vi "NXT the tug main.vi"() -> ()   [LabVIEW 2012, in "ENGR3390 Tug Boat.lvrbt"]
uses:
  ENGR3390 Tug Boat.lvrbt
  <vilib>/NXT/Block Support/NXT_InputPort.ctl
  <vilib>/NXT/Dual Mode Library/Display/drawText.vi
  <vilib>/NXT/Dual Mode Library/Sound/Tone.vi
panel:
  out "End\nIndex":i32=9
  out "Start\nIndex":i32=6
  out "Dist Array":i16[](array[numeric])
  out "IR Index":u16
  out "Dist":i16
  out "error out":errorcluster
  out "FB array":i16[](array[numeric])=[7, 8, 6, 9, 5, 10, 4, 11, 3, 12, 2, 13, 1, 14, 0, 15]
  out "Tug A":i16[](array[numeric])=[7, 8, 6, 9, 5, 10, 4, 11, 3, 12, 2, 13, 1, 14, 0, 15]
  out "FB V":i16
  out "FB H":i16
  out "Mode":i16
  out "String from PC":string
  out "Return":string
  out "Motor":u16
  out "Rudder":u16
  out "Bvolts":i32
  in  "stop":bool
  # "This is the main vi for the tug NXT code."
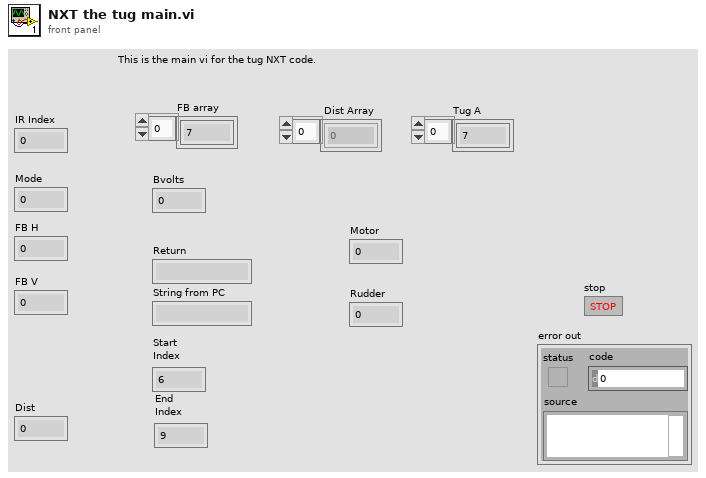
[diagram p1: front panel]
types:
  T1 = cluster{"Servo Number":u8, "Position":u16, "Speed":u8}
  T2 = typedef "NXT_InputPort.ctl" = u8
  T3 = typedef "LVHSConnector.ctl" = cluster{"Hardware":string, "Flattened String":string}
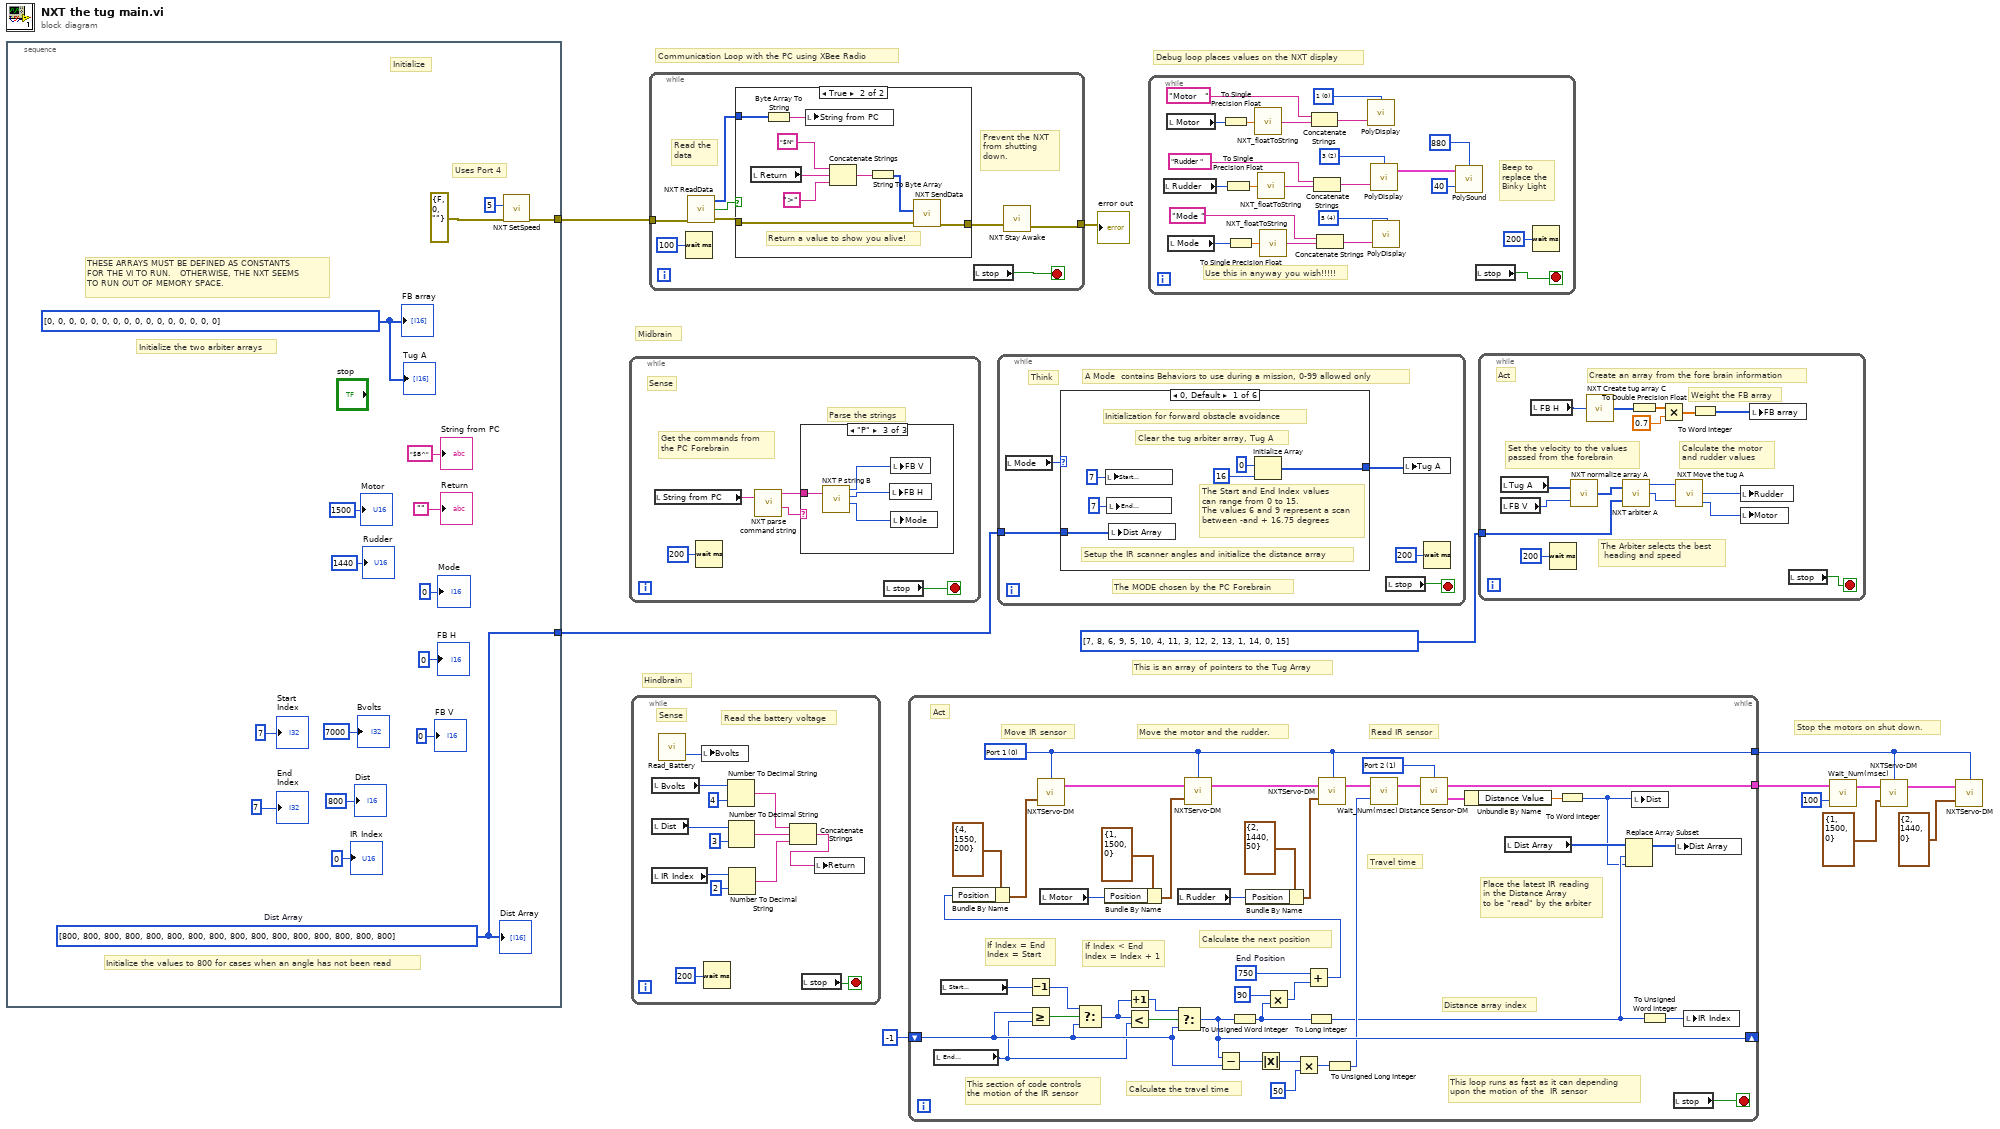
[diagram p0: block diagram]
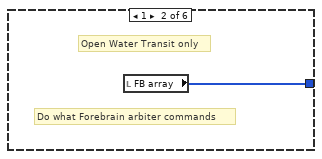
[diagram p3: hidden frame]
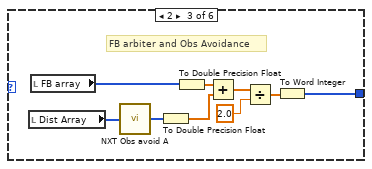
[diagram p4: hidden frame]
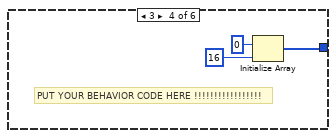
[diagram p5: hidden frame]
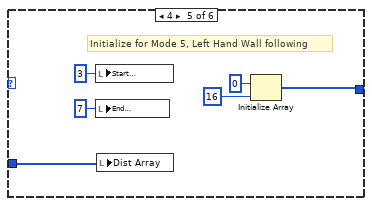
[diagram p6: hidden frame]
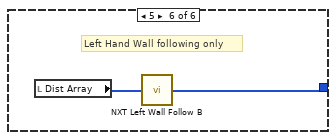
[diagram p7: hidden frame]
diagram:
  # "Debug loop places values on the NXT display"
  # "Communication Loop with the PC using XBee Radio"
  # "Stop the motors on shut down."
  # "This is an array of pointers to the Tug Array"
  # "Hindbrain"
  # "Midbrain"
  n1 = stacked-sequence {
    tunnel: [w19] -> w11
    tunnel: [w15] -> w1
    frame #0 {
      w15 = i16[] [800, 800, 800, 800, 800, 800, 800, 800, 800, 800, 800, 800, 800, 800, 800, 800]  # Dist Array
      w18 = i16[] [0, 0, 0, 0, 0, 0, 0, 0, 0, 0, 0, 0, 0, 0, 0, 0] ("Array angle\npointers")
      # "Initialize the two arbiter arrays"
      # "Initialize the values to 800 for cases when an angle has not been read"
      # "THESE ARRAYS MUST BE DEFINED AS CONSTANTS\nFOR THE VI TO RUN.   OTHERWISE, THE NXT SEEMS \nTO RUN OUT OF MEMORY SPACE."
      # "Uses Port 4"
      # "Initialize"
      n2 = call "NXT SetSpeed.vi"("error in (no error)"=errorcluster {"status"=FALSE, "code"=0, "source"=""} ("error out"), "Speed"=u8 5) -> ("error out"=w19:errorcluster)  [unwired: 5 in]
      "Bvolts" <- 7000 ("Bvolts")
      "Rudder" <- u16 1440 ("Bvolts")
      "Motor" <- u16 1500 ("Bvolts")
      "Return" <- "" ("Empty String Constant")
      "String from PC" <- "$B^" ("String from PC")
      "Mode" <- i16 0 ("Mode")
      "FB H" <- i16 0 ("Target\nHeading")
      "FB V" <- i16 0 ("Target\nHeading")
      "Tug A" <- w18
      "FB array" <- w18
      "IR Index" <- u16 0 ("IR Index")
      "Dist" <- i16 800 ("Dist")
      "Dist Array" <- w15
      "End\nIndex" <- 7 ("End\nIndex")
      "Start\nIndex" <- 7 ("Start\nIndex")
    }
  }
  n3 = while {
    stop <- w34 stop-if-true
    # "Get the commands from\nthe PC Forebrain"
    # "Parse the strings"
    # "Sense"
    n4 = local read "String from PC"() -> (w33:string)
    n5 = Wait (ms)(milliseconds to wait=u32 200) -> ()  [unwired: 1 out]
    n6 = call "NXT parse command string.vi"("String"=w33) -> ("Remaining\nString"=w31:string, "Command"=w32:string)  [unwired: 1 in, 2 out]
    n7 = case shown="\"P\"" w32 {
      tunnel: w31 -> [_ _ w35]
      frame Default {
      }
      frame "B" {
        # "Do nothing"
      }
      frame "P" {
        n8 = call "NXT P string B.vi"("string"=w35) -> ("Desired Velocity"=w38:i16, "Local Heading"=w37:i16, "Mode"=w36:i16)  [unwired: 1 in, 1 out]
        n9 = local write "FB H"(w37) -> ()
        n10 = local write "FB V"(w38) -> ()
        n11 = local write "Mode"(w36) -> ()
      }
    }
    n12 = local read "stop"() -> (w34:bool)
  }
  n13 = while {
    stop <- w51 stop-if-true
    # "Read the battery voltage"
    # "Sense"
    n14 = local read "Bvolts"() -> (w47:i32)
    n15 = local read "Dist"() -> (w46:i16)
    n16 = local read "IR Index"() -> (w44:u16)
    n17 = call <vilib>:"Read_Battery.vi"() -> ("millivolts"=w50:i32)  [unwired: 3 in, 1 out]
    n18 = local write "Bvolts"(w50) -> ()
    n19 = Wait (ms)(milliseconds to wait=u32 200) -> ()  [unwired: 1 out]
    n20 = Number To Decimal String(number=w47, width (-)=i16 4) -> (decimal integer string=w41:string)
    n21 = Number To Decimal String(number=w46, width (-)=i16 3) -> (decimal integer string=w42:string)
    n22 = Number To Decimal String(number=w44, width (-)=i16 2) -> (decimal integer string=w40:string)
    n23 = Concatenate Strings(w41, w42, w40) -> (w39:string)
    n24 = local read "stop"() -> (w51:bool)
    n25 = local write "Return"(w39) -> ()
  }
  n26 = while {
    tunnel: w11 -> [w58]
    tunnel: [w52] -> w10
    stop <- w56 stop-if-true
    # "Prevent the NXT\nfrom shutting \ndown."
    # "Read the \ndata"
    n27 = Wait (ms)(milliseconds to wait=u32 100) -> ()  [unwired: 1 out]
    n28 = call "NXT ReadData.vi"("error in (no error)"=w58) -> ("error out"=w59:errorcluster, "Valid String?"=w57:bool, "Data Out"=w55:u8[])  [unwired: 3 in]
    n29 = case shown="True" w57 {
      tunnel: [w60 w63] -> w53
      tunnel: w59 -> [w60 w68]
      tunnel: w55 -> [_ w61]
      frame False {
        # "Data is not valid\ndo nothing"
      }
      frame True {
        # "Return a value to show you alive!"
        n30 = local read "Return"() -> (w64:string)
        n31 = Byte Array To String(unsigned byte array=w61) -> (string=w62:string)
        n32 = local write "String from PC"(w62) -> ()
        n33 = Concatenate Strings("$N" ("string"), w64, ">" ("string")) -> (w65:string)
        n34 = String To Byte Array(string=w65) -> (unsigned byte array=w69:u8[])
        n35 = call "NXT SendData.vi"("error in (no error)"=w68, "Data"=w69) -> ("error out"=w63:errorcluster)  [unwired: 7 in]
      }
    }
    n36 = local read "stop"() -> (w56:bool)
    n37 = call "NXT Stay Awake.vi"("error in (no error)"=w53) -> ("error out"=w52:errorcluster)  [unwired: 2 in]
  }
  "error out" <- w10
  n38 = while {
    shift-right: [w87] -> _
    shift-left: -1 -> [w88]
    tunnel: [w80] -> w5
    tunnel: [w81] -> w4
    stop <- w104 stop-if-true
    w93 = u16 750  # End Position
    w100 = T2 1 items=["Port 1", "Port 2", "Port 3", "Port 4"] ("Input Port")
    w81 = T2 0 items=["Port 1", "Port 2", "Port 3", "Port 4"] ("Input Port")
    # "Place the latest IR reading\nin the Distance Array\nto be \"read\" by the arbiter"
    # "Distance array index"
    # "This loop runs as fast as it can depending\nupon the motion of the  IR sensor"
    # "Travel time"
    # "This section of code controls\nthe motion of the IR sensor"
    # "Calculate the next position"
    # "Calculate the travel time"
    # "If Index = End\nIndex = Start"
    # "If Index < End\nIndex = Index + 1"
    # "Read IR sensor"
    # "Move IR sensor"
    # "Move the motor and the rudder."
    # "Act"
    n39 = local read "End\nIndex"() -> (w73:i32)
    n40 = local read "Start\nIndex"() -> (w74:i32)
    n41 = Decrement(x=w74) -> (x-1=w75:i32)
    n42 = Greater Or Equal?(x=w88, y=w73) -> (x >= y?=w91:bool)
    n43 = local read "Motor"() -> (w105:u16)
    n44 = Select(t=w75, s=w91, f=w88) -> (s? t:f=w92:i32)
    n45 = Bundle By Name(cluster=T1 {"Servo Number"=1, "Position"=1500, "Speed"=0} ("Input of NXTServo"), "Position"=w105) -> (w108:T1)
    n46 = Increment(x=w92) -> (x+1=w89:i32)
    n47 = Less?(x=w92, y=w73) -> (x < y?=w90:bool)
    n48 = Select(t=w89, s=w90, f=w88) -> (s? t:f=w87:i32)
    n49 = local read "Rudder"() -> (w106:u16)
    n50 = Subtract(x=w87, y=w88) -> (x-y=w96:i32)
    n51 = To Unsigned Word Integer(number=w87) -> (unsigned 16bit integer=w79:u16)
    n52 = Bundle By Name(cluster=T1 {"Servo Number"=2, "Position"=1440, "Speed"=50} ("Input of NXTServo"), "Position"=w106) -> (w111:T1)
    n53 = Absolute Value(x=w96) -> (abs(x)=w97:i32)
    n54 = Multiply(x=u16 90, y=w79) -> (x*y=w95:u16)
    n55 = Multiply(x=w97, y=50) -> (x*y=w84:i32)
    n56 = Add(x=w93, y=w95) -> (x+y=w82:u16)
    n57 = Bundle By Name(cluster=T1 {"Servo Number"=4, "Position"=1550, "Speed"=200} ("Input of NXTServo"), "Position"=w82) -> (w103:T1)
    n58 = call "NXTServo-DM.vi"("Input of NXTServo"=w103, "Input Port"=w81) -> ("NXT dup"=w101:T3)  [unwired: 1 in, 1 out]
    n59 = call "NXTServo-DM.vi"("Input of NXTServo"=w108, "NXT"=w101, "Input Port"=w81) -> ("NXT dup"=w107:T3)  [unwired: 1 out]
    n60 = To Long Integer(number=w79) -> (32bit integer=w72:i32)
    n61 = call "NXTServo-DM.vi"("Input of NXTServo"=w111, "NXT"=w107, "Input Port"=w81) -> ("NXT dup"=w86:T3)  [unwired: 1 out]
    n62 = To Unsigned Long Integer(number=w84) -> (unsigned 32bit integer=w83:u32)
    n63 = call <vilib>:"Wait_Num(msec).vi"("Time (100 msec)"=w83, "NXT"=w86) -> ("NXT"=w85:T3)  [unwired: 2 in]
    n64 = call "Distance Sensor-DM.vi"("NXT"=w85, "Input Port"=w100) -> ("Output of Distance Sensor"=w99:cluster{"Distance Value":ext, "Status":bool}, "NXT dup"=w80:T3)  [unwired: 1 in]
    n65 = Unbundle By Name(w99) -> ("Distance Value"=w78:ext)
    n66 = local read "Dist Array"() -> (w77:i16[])
    n67 = To Word Integer(number=w78) -> (16bit integer=w70:i16)
    n68 = Replace Array Subset(array=w77, new element=w70, index=w72) -> (w76:i16[])
    n69 = local write "Dist"(w70) -> ()
    n70 = To Unsigned Word Integer(number=w72) -> (unsigned 16bit integer=w71:u16)
    n71 = local read "stop"() -> (w104:bool)
    n72 = local write "Dist Array"(w76) -> ()
    n73 = local write "IR Index"(w71) -> ()
  }
  n74 = while {
    tunnel: w1 -> [w112]
    stop <- w116 stop-if-true
    # "The MODE chosen by the PC Forebrain"
    # "A Mode  contains Behaviors to use during a mission, 0-99 allowed only"
    # "Think"
    n75 = local read "Mode"() -> (w115:i16)
    n76 = case shown="0, Default" w115 {
      tunnel: [w120 w123 w125 w133 w136 w142] -> w114
      tunnel: w112 -> [w119 _ _ _ w139 _]
      frame 0, Default {
        # "The Start and End Index values \ncan range from 0 to 15.\nThe values 6 and 9 represent a scan\nbetween -and + 16.75 degrees"
        # "Setup the IR scanner angles and initialize the distance array"
        # "Clear the tug arbiter array, Tug A"
        # "Initialization for forward obstacle avoidance"
        n77 = local write "Start\nIndex"(7 ("Start\nIndex")) -> ()
        n78 = local write "End\nIndex"(7 ("End\nIndex")) -> ()
        n79 = local write "Dist Array"(w119) -> ()
        n80 = Initialize Array(i16 0 ("element"), 16 ("dimension size")) -> (w120:i16[])
      }
      frame 1 {
        # "Open Water Transit only"
        # "Do what Forebrain arbiter commands"
        n81 = local read "FB array"() -> (w123:i16[])
      }
      frame 2 {
        # "FB arbiter and Obs Avoidance"
        n82 = local read "Dist Array"() -> (w124:i16[])
        n83 = local read "FB array"() -> (w128:i16[])
        n84 = call "NXT Obs avoid A.vi"("Distance array"=w124) -> ("Obs array"=w127:i16[])
        n85 = To Double Precision Float(number=w127) -> (double precision float=w126:dbl[])
        n86 = To Double Precision Float(number=w128) -> (double precision float=w132:dbl[])
        n87 = Add(x=w132, y=w126) -> (x+y=w131:dbl[])
        n88 = Divide(x=w131, y=2.0) -> (x/y=w129:dbl[])
        n89 = To Word Integer(number=w129) -> (16bit integer=w125:i16[])
      }
      frame 3 {
        # "PUT YOUR BEHAVIOR CODE HERE !!!!!!!!!!!!!!!!!"
        n90 = Initialize Array(i16 0 ("element"), 16 ("dimension size")) -> (w133:i16[])
      }
      frame 4 {
        # "Initialize for Mode 5, Left Hand Wall following"
        n91 = local write "Start\nIndex"(3 ("Start\nIndex")) -> ()
        n92 = local write "End\nIndex"(7 ("End\nIndex")) -> ()
        n93 = local write "Dist Array"(w139) -> ()
        n94 = Initialize Array(i16 0 ("element"), 16 ("dimension size")) -> (w136:i16[])
      }
      frame 5 {
        # "Left Hand Wall following only"
        n95 = local read "Dist Array"() -> (w143:i16[])
        n96 = call "NXT Left Wall Follow B.vi"("Distance array"=w143) -> ("ouput array"=w142:i16[])
      }
    }
    n97 = local read "stop"() -> (w116:bool)
    n98 = local write "Tug A"(w114) -> ()
    n99 = Wait (ms)(milliseconds to wait=u32 200) -> ()  [unwired: 1 out]
  }
  n100 = while {
    stop <- w166 stop-if-true
    w150 = i16 4 items=["1", "2", "3", "4", "5", "6", "7", "8"] ("Line")
    w156 = i16 2 items=["1", "2", "3", "4", "5", "6", "7", "8"] ("Line")
    w160 = i16 0 items=["1", "2", "3", "4", "5", "6", "7", "8"] ("Line")
    # "Use this in anyway you wish!!!!!"
    # "Beep to \nreplace the\nBinky Light"
    n101 = local read "Rudder"() -> (w154:u16)
    n102 = local read "Motor"() -> (w165:u16)
    n103 = local read "Mode"() -> (w149:i16)
    n104 = To Single Precision Float(number=w165) -> (single precision float=w164:sgl)
    n105 = To Single Precision Float(number=w154) -> (single precision float=w157:sgl)
    n106 = To Single Precision Float(number=w149) -> (single precision float=w151:sgl)
    n107 = call <vilib>:"NXT_floatToString.vi"("number"=w164) -> ("string"=w162:string)
    n108 = call <vilib>:"NXT_floatToString.vi"("number"=w157) -> ("string"=w158:string)
    n109 = call <vilib>:"NXT_floatToString.vi"("number"=w151) -> ("string"=w152:string)
    n110 = Concatenate Strings("Motor   ", w162) -> (w161:string)
    n111 = Concatenate Strings("Rudder ", w158) -> (w159:string)
    n112 = Concatenate Strings("Mode ", w152) -> (w153:string)
    n113 = call-poly <vilib>:"PolyDisplay.vi"("Text"=w161, "Line"=w160) -> ()  [unwired: 2 in, 1 out]
    n114 = call-poly <vilib>:"PolyDisplay.vi"("Text"=w159, "Line"=w156) -> ("NXT"=w145:T3)  [unwired: 2 in]
    n115 = call-poly <vilib>:"PolyDisplay.vi"("Text"=w153, "Line"=w150) -> ()  [unwired: 2 in, 1 out]
    n116 = call-poly <vilib>:"PolySound.vi"("Duration (500 ms)"=u16 40, "NXT"=w145, "Tone (440 Hz)"=u16 880) -> ()  [unwired: 1 in, 1 out]
    n117 = local read "stop"() -> (w166:bool)
    n118 = Wait (ms)(milliseconds to wait=u32 200) -> ()  [unwired: 1 out]
  }
  n119 = while {
    tunnel: i16[] [7, 8, 6, 9, 5, 10, 4, 11, 3, 12, 2, 13, 1, 14, 0, 15] ("Array angle\npointers") -> [w177]
    stop <- w182 stop-if-true
    # "Create an array from the fore brain information"
    # "Calculate the motor\nand rudder values"
    # "Set the velocity to the values\npassed from the forebrain"
    # "Weight the FB array"
    # "The Arbiter selects the best\n heading and speed"
    # "Act"
    n120 = local read "Tug A"() -> (w169:i16[])
    n121 = local read "FB V"() -> (w168:i16)
    n122 = local read "FB H"() -> (w179:i16)
    n123 = Wait (ms)(milliseconds to wait=u32 200) -> ()  [unwired: 1 out]
    n124 = call "NXT normalize array A.vi"("FB Arbiter\nVelocity"=w168, "Tug array"=w169) -> ("Normalized\nArray"=w167:i16[])
    n125 = call "NXT Create tug array C.vi"("Local Heading"=w179) -> ("FB array"=w171:i16[])  [unwired: 2 in]
    n126 = call "NXT arbiter A.vi"("Tug array"=w167, "Array angle\npointers"=w177) -> ("Arbiter Heading"=w176:i16, "Arbiter\nvelocity"=w175:i16)  [unwired: 1 out]
    n127 = To Double Precision Float(number=w171) -> (double precision float=w174:dbl[])
    n128 = Multiply(x=w174, y=0.7 ("FB weight")) -> (x*y=w173:dbl[])
    n129 = call "NXT Move the tug A.vi"("Arbiter Heading"=w176, "Desired Speed"=w175) -> ("Rudder"=w181:u16, "Motor"=w180:u16)  [unwired: 1 out]
    n130 = To Word Integer(number=w173) -> (16bit integer=w170:i16[])
    n131 = local write "Rudder"(w181) -> ()
    n132 = local write "Motor"(w180) -> ()
    n133 = local write "FB array"(w170) -> ()
    n134 = local read "stop"() -> (w182:bool)
  }
  n135 = call <vilib>:"Wait_Num(msec).vi"("Time (100 msec)"=u32 100, "NXT"=w5) -> ("NXT"=w6:T3)  [unwired: 2 in]
  n136 = call "NXTServo-DM.vi"("Input of NXTServo"=T1 {"Servo Number"=1, "Position"=1500, "Speed"=0}, "NXT"=w6, "Input Port"=w4) -> ("NXT dup"=w9:T3)  [unwired: 1 out]
  n137 = call "NXTServo-DM.vi"("Input of NXTServo"=T1 {"Servo Number"=2, "Position"=1440, "Speed"=0}, "NXT"=w9, "Input Port"=w4) -> ()  [unwired: 2 out]
